vi "Auto-Home_Startup.vi"(1 "Enabled?":bool, 2 "Enum":T1) -> (0 "Activate_Auto-Home":bool)   [LabVIEW 2019]
uses:
  TypeDefs/Hood_Homing_State.ctl
  ArgosLib/ArgosLib.lvlib
  ArgosLib/Signal Processing/TypeDefs/EdgeDetector_Type.ctl
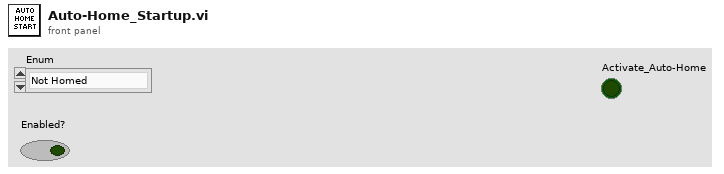
[diagram p1: front panel]
types:
  T1 = typedef "Hood_Homing_State.ctl" = enum16{"Not Homed", "Homing in Process", "Homing Failed", "Homing Completed"}
  T2 = typedef "ArgosLib.lvlib/EdgeDetector_Type.ctl" = enum16{"RisingEdge", "FallingEdge", "Both"}
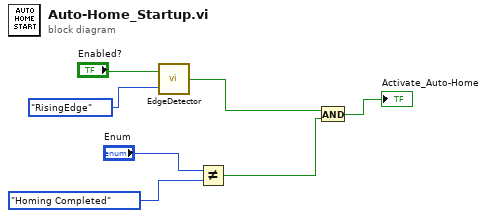
[diagram p0: block diagram]
diagram:
  n1 = call "EdgeDetector.vi"("DetectorType"=EdgeDetector_Type."RisingEdge", "Input"="Enabled?") -> ("Edge"=w2:bool)
  n2 = Not Equal?(x="Enum", y=Hood_Homing_State."Homing Completed" ("Enum")) -> (x != y?=w4:bool)
  n3 = And(x=w2, y=w4) -> (x .and. y?=→"Activate_Auto-Home":bool)
